vi "HandleInput.vi"(8 "error in (no error)":errorcluster, 11 "TeleopInstruction":T1) -> (0 "error out":errorcluster)   [LabVIEW 2013]
uses:
  TeleopInstruction.ctl
  DriveInstruction.ctl
  QueueSubsystem.ctl
  QueueAction.ctl
panel:
  in  "Deadzone":dbl=0.1
  out "Time":u32
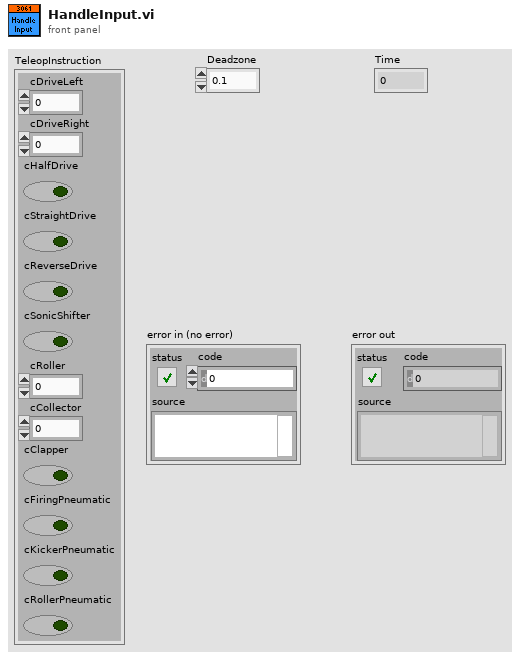
[diagram p1: front panel]
types:
  T1 = typedef "TeleopInstruction.ctl" = cluster{"cDriveLeft":dbl, "cDriveRight":dbl, "cHalfDrive":bool, "cStraightDrive":bool, "cReverseDrive":bool, "cSonicShifter":bool, "cRoller":dbl, "cCollector":dbl, "cClapper":bool, "cFiringPneumatic":bool, "cKickerPneumatic":bool, "cRollerPneumatic":bool}
  T2 = typedef "DriveInstruction.ctl" = cluster{"cDriveLeft":dbl, "cDriveRight":dbl, "cHalfDrive":bool, "cStraightDrive":bool, "cReverseDrive":bool}
  T3 = typedef "QueueAction.ctl" = enum16{"Init", "SetValue", "Disable"}
  T4 = typedef "QueueSubsystem.ctl" = enum16{"Drive", "SonicShifter", "Kicker", "FirePneumatic", "Roller", "Clapper", "RollerRelay"}
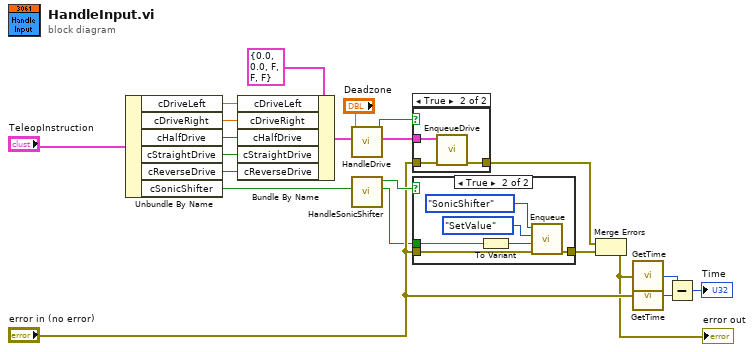
[diagram p0: block diagram]
diagram:
  n1 = Unbundle By Name("TeleopInstruction") -> ("cDriveLeft"=w11:dbl, "cDriveRight"=w10:dbl, "cHalfDrive"=w14:bool, "cStraightDrive"=w13:bool, "cReverseDrive"=w12:bool, "cSonicShifter"=w2:bool)
  n2 = Bundle By Name(cluster=T2 {"cDriveLeft"=0.0, "cDriveRight"=0.0, "cHalfDrive"=FALSE, "cStraightDrive"=FALSE, "cReverseDrive"=FALSE} ("DriveInstruction"), "cDriveLeft"=w11, "cDriveRight"=w10, "cHalfDrive"=w14, "cStraightDrive"=w13, "cReverseDrive"=w12) -> (w8:T2)
  n3 = call "HandleDrive.vi"("DriveInstruction"=w8, "Deadzone"="Deadzone") -> ("DriveInstruction"=w9:T2, "Enqueue?"=w16:bool)  [unwired: 8 in]
  n4 = call "HandleSonicShifter.vi"("cSonicShifter"=w2) -> ("cSonicShifter"=w1:bool, "Enqueue?"=w7:bool)  [unwired: 9 in]
  n5 = case shown="True" w16 {
    tunnel: [w22 w25] -> w5
    tunnel: "error in (no error)" -> [w22 w24]
    tunnel: w9 -> [_ w23]
    frame False {
    }
    frame True {
      n6 = call "EnqueueDrive.vi"("error in (no error)"=w24, "DriveInstruction"=w23) -> ("error out"=w25:errorcluster)  [unwired: 9 in]
    }
  }
  n7 = case shown="True" w7 {
    tunnel: "error in (no error)" -> [w26 w32]
    tunnel: [w26 w31] -> w4
    tunnel: w1 -> [_ w27]
    frame False {
    }
    frame True {
      n8 = To Variant(anything=w27) -> (Variant=w28:variant)
      n9 = call "Enqueue.vi"("error in (no error)"=w32, "Data"=w28, "Action"=QueueAction."SetValue", "Subsystem"=QueueSubsystem."SonicShifter") -> ("error out"=w31:errorcluster)  [unwired: 7 in]
    }
  }
  n10 = Merge Errors(w5, w4) -> (w3:errorcluster)
  "error out" <- w3
  n11 = call "GetTime.vi"("error in"=w3) -> ("Time"=w20:u32)
  n12 = call "GetTime.vi"("error in"="error in (no error)") -> ("Time"=w19:u32)
  n13 = Subtract(x=w20, y=w19) -> (x-y=→"Time":u32)
